vi "Update Normalized Axes.vi"(8 "axis in":T2, 11 "Device in":T1={"device ID"=refnum, "Device Name"="Logitech Extreme 3D", "axis info"={"X axis"=[], "Y axis"=[], "Z axis"=[], "X axis rotation"=[], "Y axis rotation"=[], "Z axis rotation"=[], "U axis"=[], "V axis"=[]}}) -> (0 "axis out":T2, 3 "Device out":T1={"device ID"=refnum, "Device Name"="Logitech Extreme 3D", "axis info"={"X axis"=[], "Y axis"=[], "Z axis"=[], "X axis rotation"=[], "Y axis rotation"=[], "Z axis rotation"=[], "U axis"=[], "V axis"=[]}})   [LabVIEW 2012]
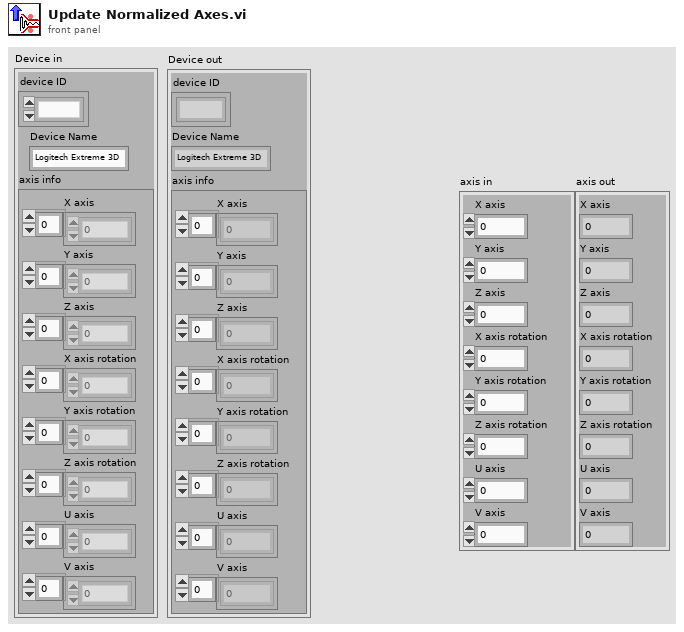
[diagram p1: front panel]
types:
  T1 = cluster{"device ID":refnum<k1>, "Device Name":string, "axis info":cluster{"X axis":dbl[], "Y axis":dbl[], "Z axis":dbl[], "X axis rotation":dbl[], "Y axis rotation":dbl[], "Z axis rotation":dbl[], "U axis":dbl[], "V axis":dbl[]}}
  T2 = cluster{"X axis":i32, "Y axis":i32, "Z axis":i32, "X axis rotation":i32, "Y axis rotation":i32, "Z axis rotation":i32, "U axis":i32, "V axis":i32}
  T3 = cluster{"X axis":dbl[], "Y axis":dbl[], "Z axis":dbl[], "X axis rotation":dbl[], "Y axis rotation":dbl[], "Z axis rotation":dbl[], "U axis":dbl[], "V axis":dbl[]}
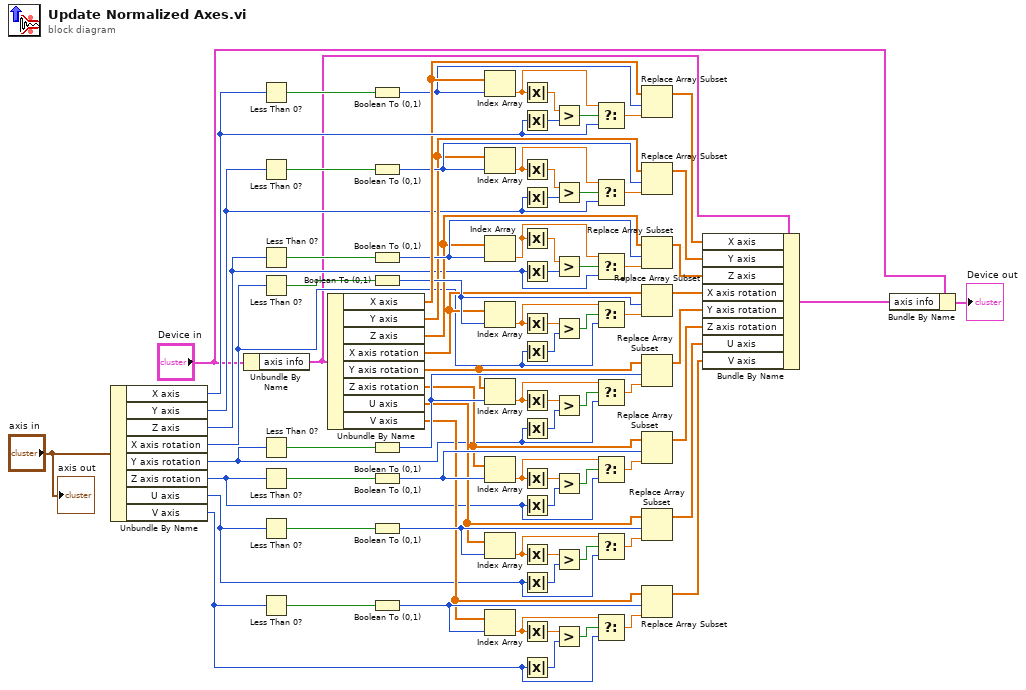
[diagram p0: block diagram]
diagram:
  n1 = Unbundle By Name("axis in") -> ("X axis"=w80:i32, "Y axis"=w11:i32, "Z axis"=w10:i32, "X axis rotation"=w9:i32, "Y axis rotation"=w8:i32, "Z axis rotation"=w7:i32, "U axis"=w6:i32, "V axis"=w5:i32)
  n2 = Unbundle By Name("Device in") -> ("axis info"=w1:T3)
  n3 = Less Than 0?(x=w80) -> (x < 0?=w85:bool)
  n4 = Less Than 0?(x=w11) -> (x < 0?=w69:bool)
  n5 = Less Than 0?(x=w10) -> (x < 0?=w68:bool)
  n6 = Less Than 0?(x=w9) -> (x < 0?=w55:bool)
  n7 = Less Than 0?(x=w8) -> (x < 0?=w54:bool)
  n8 = Less Than 0?(x=w7) -> (x < 0?=w41:bool)
  n9 = Less Than 0?(x=w6) -> (x < 0?=w40:bool)
  n10 = Less Than 0?(x=w5) -> (x < 0?=w20:bool)
  n11 = Unbundle By Name(w1) -> ("X axis"=w79:dbl[], "Y axis"=w18:dbl[], "Z axis"=w17:dbl[], "X axis rotation"=w16:dbl[], "Y axis rotation"=w15:dbl[], "Z axis rotation"=w14:dbl[], "U axis"=w13:dbl[], "V axis"=w12:dbl[])
  n12 = Boolean To (0,1)(Boolean=w85) -> (0, 1=w78:i16)
  n13 = Boolean To (0,1)(Boolean=w69) -> (0, 1=w74:i16)
  n14 = Boolean To (0,1)(Boolean=w68) -> (0, 1=w63:i16)
  n15 = Boolean To (0,1)(Boolean=w55) -> (0, 1=w60:i16)
  n16 = Boolean To (0,1)(Boolean=w54) -> (0, 1=w49:i16)
  n17 = Boolean To (0,1)(Boolean=w41) -> (0, 1=w46:i16)
  n18 = Boolean To (0,1)(Boolean=w40) -> (0, 1=w35:i16)
  n19 = Boolean To (0,1)(Boolean=w20) -> (0, 1=w25:i16)
  n20 = Index Array(array=w79, index=w78) -> (element=w81:dbl)
  n21 = Index Array(array=w18, index=w74) -> (element=w73:dbl)
  n22 = Index Array(array=w17, index=w63) -> (element=w64:dbl)
  n23 = Index Array(array=w16, index=w60) -> (element=w59:dbl)
  n24 = Index Array(array=w15, index=w49) -> (element=w50:dbl)
  n25 = Index Array(array=w14, index=w46) -> (element=w45:dbl)
  n26 = Index Array(array=w13, index=w35) -> (element=w36:dbl)
  n27 = Index Array(array=w12, index=w25) -> (element=w24:dbl)
  n28 = Absolute Value(x=w81) -> (abs(x)=w83:dbl)
  n29 = Absolute Value(x=w80) -> (abs(x)=w82:i32)
  n30 = Absolute Value(x=w73) -> (abs(x)=w71:dbl)
  n31 = Absolute Value(x=w11) -> (abs(x)=w72:i32)
  n32 = Absolute Value(x=w64) -> (abs(x)=w66:dbl)
  n33 = Absolute Value(x=w10) -> (abs(x)=w65:i32)
  n34 = Absolute Value(x=w59) -> (abs(x)=w57:dbl)
  n35 = Absolute Value(x=w9) -> (abs(x)=w58:i32)
  n36 = Absolute Value(x=w50) -> (abs(x)=w52:dbl)
  n37 = Absolute Value(x=w8) -> (abs(x)=w51:i32)
  n38 = Absolute Value(x=w45) -> (abs(x)=w43:dbl)
  n39 = Absolute Value(x=w7) -> (abs(x)=w44:i32)
  n40 = Absolute Value(x=w36) -> (abs(x)=w38:dbl)
  n41 = Absolute Value(x=w6) -> (abs(x)=w37:i32)
  n42 = Absolute Value(x=w24) -> (abs(x)=w22:dbl)
  n43 = Absolute Value(x=w5) -> (abs(x)=w23:i32)
  n44 = Greater?(x=w83, y=w82) -> (0:w84:bool)
  n45 = Greater?(x=w71, y=w72) -> (0:w70:bool)
  n46 = Greater?(x=w66, y=w65) -> (0:w67:bool)
  n47 = Greater?(x=w57, y=w58) -> (0:w56:bool)
  n48 = Greater?(x=w52, y=w51) -> (0:w53:bool)
  n49 = Greater?(x=w43, y=w44) -> (0:w42:bool)
  n50 = Greater?(x=w38, y=w37) -> (0:w39:bool)
  n51 = Greater?(x=w22, y=w23) -> (0:w21:bool)
  n52 = Select(t=w81, s=w84, f=w80) -> (s? t:f=w77:dbl)
  n53 = Select(t=w73, s=w70, f=w11) -> (s? t:f=w75:dbl)
  n54 = Select(t=w64, s=w67, f=w10) -> (s? t:f=w62:dbl)
  n55 = Select(t=w59, s=w56, f=w9) -> (s? t:f=w61:dbl)
  n56 = Select(t=w50, s=w53, f=w8) -> (s? t:f=w48:dbl)
  n57 = Select(t=w45, s=w42, f=w7) -> (s? t:f=w47:dbl)
  n58 = Select(t=w36, s=w39, f=w6) -> (s? t:f=w34:dbl)
  n59 = Select(t=w24, s=w21, f=w5) -> (s? t:f=w26:dbl)
  n60 = Replace Array Subset(array=w79, new element=w77, index=w78) -> (w33:dbl[])
  n61 = Replace Array Subset(array=w18, new element=w75, index=w74) -> (w32:dbl[])
  n62 = Replace Array Subset(array=w17, new element=w62, index=w63) -> (w31:dbl[])
  n63 = Replace Array Subset(array=w16, new element=w61, index=w60) -> (w30:dbl[])
  n64 = Replace Array Subset(array=w15, new element=w48, index=w49) -> (w29:dbl[])
  n65 = Replace Array Subset(array=w14, new element=w47, index=w46) -> (w28:dbl[])
  n66 = Replace Array Subset(array=w13, new element=w34, index=w35) -> (w27:dbl[])
  n67 = Replace Array Subset(array=w12, new element=w26, index=w25) -> (w19:dbl[])
  n68 = Bundle By Name(cluster=w1, "X axis"=w33, "Y axis"=w32, "Z axis"=w31, "X axis rotation"=w30, "Y axis rotation"=w29, "Z axis rotation"=w28, "U axis"=w27, "V axis"=w19) -> (w2:T3)
  n69 = Bundle By Name(cluster="Device in", "axis info"=w2) -> (→"Device out":T1)
  "axis out" <- "axis in"
